vi "UI_多电机初始化模块.vi"(5 "压电默认位置":dbl, 7 "device index输入":T1, 8 "错误输入（无错误）":errorcluster, 9 "piezo pos":refnum<vi>, 10 "mg rot":refnum<vi>, 11 "mg pos":refnum<vi>) -> (0 "错误输出":errorcluster, 3 "device index输出":T1)   [LabVIEW 2017]
uses:
  device index.ctl
  labview setup procedure.ctl
  velocity set control.ctl
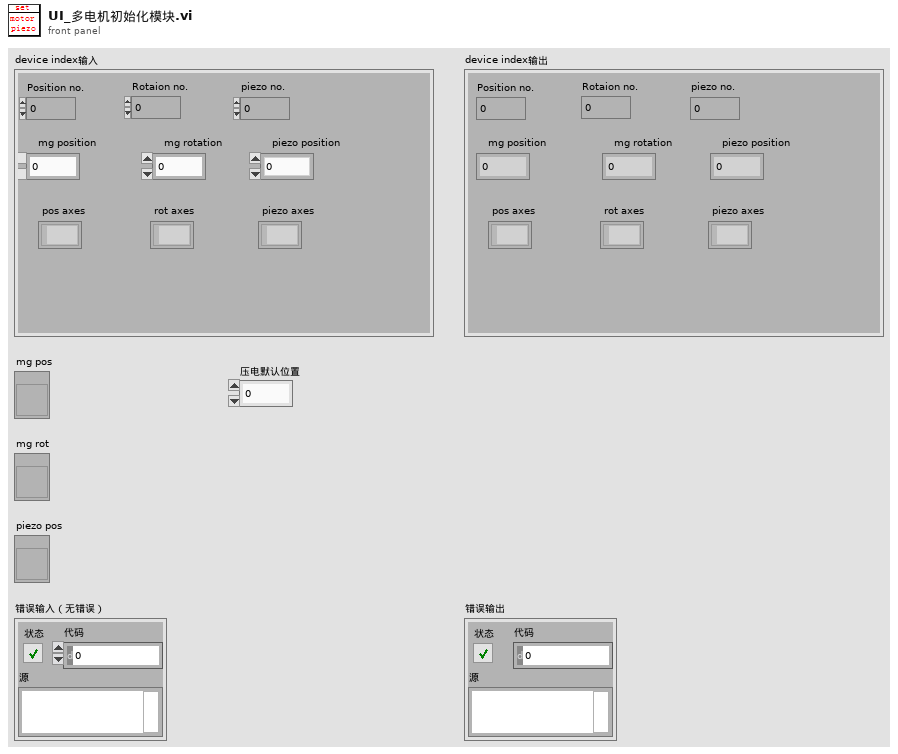
[diagram p1: front panel]
types:
  T1 = typedef "device index.ctl" = cluster{"Position no.":i32, "Rotaion no.":i32, "piezo no.":i32, "mg position":dbl, "mg rotation":dbl, "piezo position":dbl, "pos axes":string[], "rot axes":string[], "piezo axes":string[]}
  T2 = typedef "labview setup procedure.ctl" = enum16{"仪器注销", "注册并校准仪器", "设置仪器速度", "完成设置", "清除ROI", "结束磁铁循环"}
  T3 = typedef "velocity set control.ctl" = cluster{"平移电机速度":dbl, "旋转电机速度":dbl}
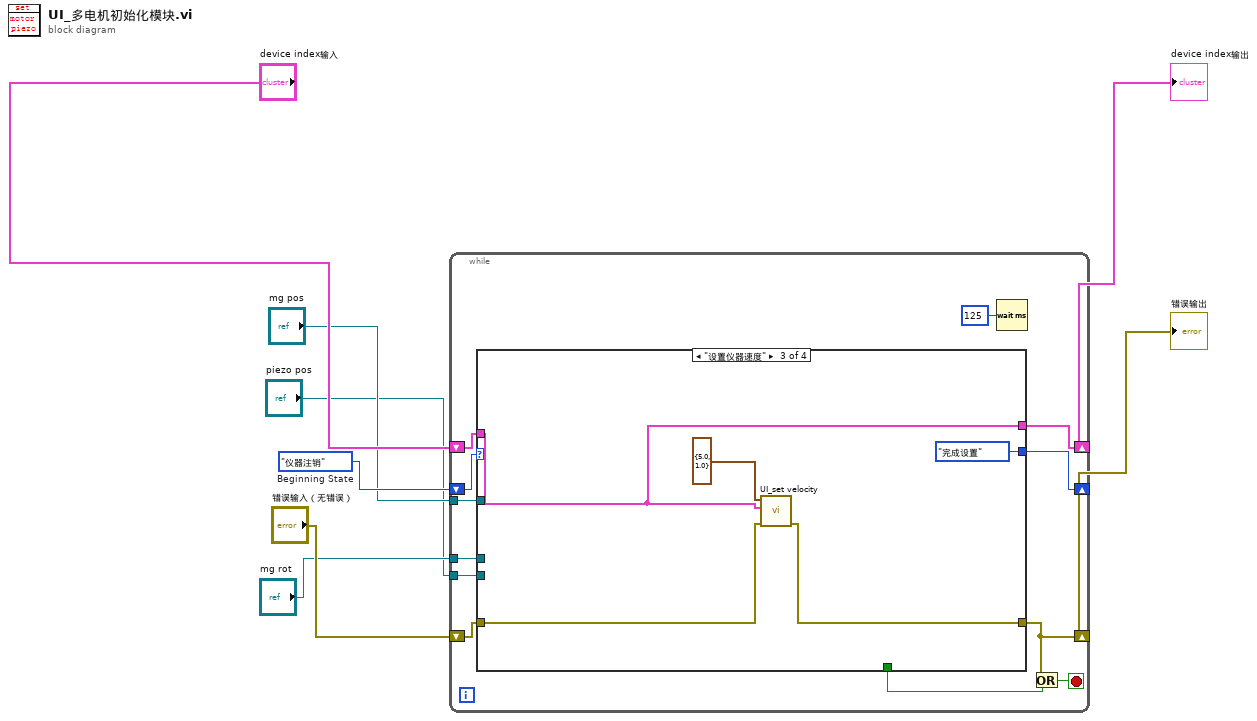
[diagram p0: block diagram]
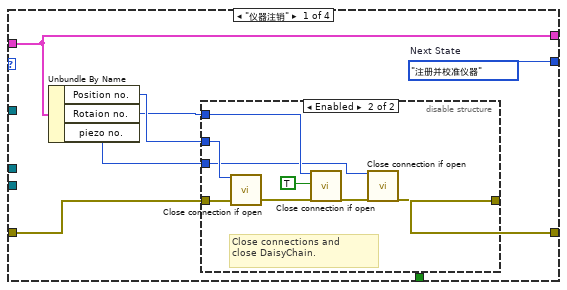
[diagram p2: hidden frame]
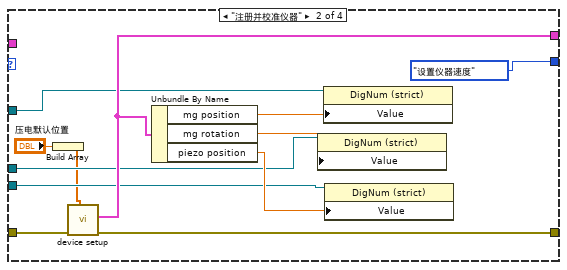
[diagram p4: hidden frame]
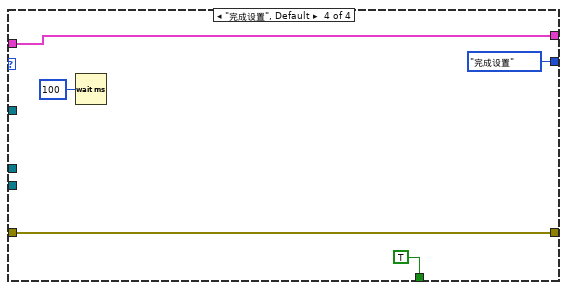
[diagram p5: hidden frame]
diagram:
  w4 = labview_setup_procedure."仪器注销"  # Beginning State
  n1 = while {
    shift-right: [w19] -> _
    shift-left: w4 -> [w20]
    shift-right: [w15] -> w8
    shift-left: "device index输入" -> [w17]
    shift-right: [w14] -> w6
    shift-left: "错误输入（无错误）" -> [w16]
    tunnel: "mg pos" -> [w11]
    tunnel: "mg rot" -> [w10]
    tunnel: "piezo pos" -> [w9]
    stop <- w13 stop-if-true
    n2 = case shown="\"设置仪器速度\"" w20 {
      tunnel: [w27 labview_setup_procedure."设置仪器速度" ("Next State") labview_setup_procedure."完成设置" ("Next State") labview_setup_procedure."完成设置" ("Next State")] -> w19
      tunnel: w17 -> [w21 _ w50 w58]
      tunnel: w16 -> [w23 w47 w52 w55]
      tunnel: [w22 w46 w51 w55] -> w14
      tunnel: [w21 w45 w50 w58] -> w15
      tunnel: [_ _ _ TRUE] -> w12
      tunnel: w11 -> [_ w41 _ _]
      tunnel: w10 -> [_ w40 _ _]
      tunnel: w9 -> [_ w39 _ _]
      frame "仪器注销" {
        w27 = labview_setup_procedure."注册并校准仪器"  # Next State
        n3 = Unbundle By Name(w21) -> ("Position no."=w26:i32, "Rotaion no."=w25:i32, "piezo no."=w24:i32)
        n4 = disable-structure shown="Enabled" {
          disable-tunnel: w26 -> [_ w33]
          disable-tunnel: w25 -> [_ w32]
          disable-tunnel: w24 -> [_ w31]
          disable-tunnel: w23 -> [w28 w29]
          disable-tunnel: [w28 w30] -> w22
          frame Disabled {
          }
          frame Enabled {
            # "Close connections and\nclose DaisyChain."
            n5 = call "Close connection if open.vi"("System no."=w33, "error in"=w29) -> ("error out"=w34:errorcluster)  [unwired: 16 in, 1 out]
            n6 = call "Close connection if open.vi"("System no."=w32, "Close DaisyChain"=TRUE, "error in"=w34) -> ("error out"=w36:errorcluster)  [unwired: 15 in, 1 out]
            n7 = call "Close connection if open.vi"("System no."=w31, "error in"=w36) -> ("error out"=w30:errorcluster)  [unwired: 16 in, 1 out]
          }
        }
      }
      frame "注册并校准仪器" {
        n8 = Build Array("压电默认位置") -> (w37:dbl[])
        n9 = call "device setup.vi"("good pos"=w37, "error in (no error)"=w47) -> ("error out"=w46:errorcluster, "device index out"=w45:T1)  [unwired: 8 in]
        n10 = Unbundle By Name(w45) -> ("mg position"=w44:dbl, "mg rotation"=w43:dbl, "piezo position"=w42:dbl)
        n11 = property class="DigNum (strict)"(reference=w40, "Value"=w43) -> ()  [unwired: 1 in, 2 out]
        n12 = property class="DigNum (strict)"(reference=w41, "Value"=w44) -> ()  [unwired: 1 in, 2 out]
        n13 = property class="DigNum (strict)"(reference=w39, "Value"=w42) -> ()  [unwired: 1 in, 2 out]
      }
      frame "设置仪器速度" {
        n14 = call "UI_set velocity.vi"("error in (no error)"=w52, "device index"=w50, "velocity set"=T3 {"平移电机速度"=5.0, "旋转电机速度"=1.0} ("数据")) -> ("error out"=w51:errorcluster)  [unwired: 6 in, 2 out]
      }
      frame "完成设置", Default {
        n15 = Wait (ms)(milliseconds to wait=u32 100 ("等待时间（毫秒）")) -> ()  [unwired: 1 out]
      }
    }
    n16 = Wait (ms)(milliseconds to wait=u32 125) -> ()  [unwired: 1 out]
    n17 = Or(x=w14, y=w12) -> (x .or. y?=w13:bool)
  }
  "device index输出" <- w8
  "错误输出" <- w6
